vi "libssh2_keepalive_config.vi"(8 "error in (no error)":errorcluster, 9 "want reply (F)":bool, 10 "interval (0 = disabled)":u32, 11 "session":T1) -> (0 "error out":errorcluster)   [LabVIEW 2013, in "libssh2.lvlib"]
doc: "Set how often keep-alive messages should be send. <B>want reply</B> indicates whether the keep-alive messages should request a response from the server. <B>interval</B> is the number of seconds that can pass without I/O.\n\nNote that an interval of 1 will be treated as 2 by libssh2 to avoid some busy-loop corner-cases.\n\nThe caller is responsible for sending keep-alive messages using <B>libssh2_keepalive_send</B>."
uses:
  libssh2.lvlib
  Session Refnum.ctl
  Not A Session.vi
  <vilib>/Utility/error.llb/Error Cluster From Error Code.vi
  Global Settings.vi
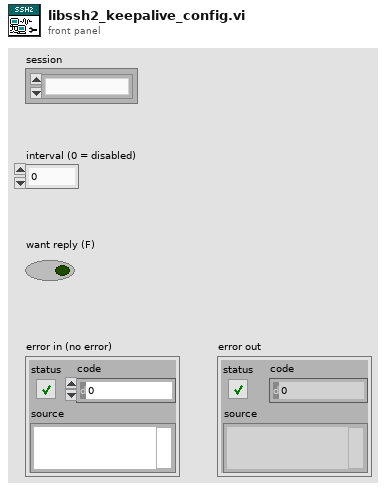
[diagram p1: front panel]
types:
  T1 = typedef "libssh2.lvlib/Session Refnum.ctl" = refnum<k1>
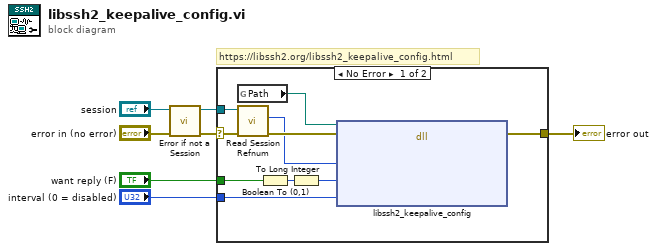
[diagram p0: block diagram]
diagram:
  # "https://libssh2.org/libssh2_keepalive_config.html"
  n1 = call "Error if not a Session.vi"("error in (no error)"="error in (no error)", "session"="session") -> ("error out"=w5:errorcluster, "session out"=w3:T1)  [unwired: 8 in]
  n2 = case shown="No Error" w5 {
    selector: w5 -> [w16 w18]
    tunnel: [w17 w18] -> w7
    tunnel: w3 -> [w15 _]
    tunnel: "interval (0 = disabled)" -> [w11 _]
    tunnel: "want reply (F)" -> [w10 _]
    frame No Error {
      n3 = global read "Global Settings.vi" "Path"() -> (w12:path)
      n4 = call "Read Session Refnum.vi"("error in (no error)"=w16, "session"=w15) -> ("error out"=w14:errorcluster, "LIBSSH2_SESSION*"=w13:u64)  [unwired: 5 in, 3 out]
      n5 = Boolean To (0,1)(Boolean=w10) -> (0, 1=w9:i16)
      n6 = To Long Integer(number=w9) -> (32bit integer=w8:i32)
      n7 = dll-call lib="?" fn="libssh2_keepalive_config"(path in=w12, error in=w14, "session"=w13, "want_reply"=w8, "interval"=w11) -> (error out=w17:errorcluster)  [unwired: 5 in, 1 out]
    }
    frame Error {
    }
  }
  "error out" <- w7
